vi "Set Settings.vi"(8 "error in (no error)":errorcluster, 10 "Settings":T1, 11 "Acrobat Template in":refnum<class "Application.lvclass">) -> (0 "error out":errorcluster, 3 "Acrobat Template out":refnum<class "Application.lvclass">)   [LabVIEW 2017, in "Application.lvlib" / "Application.lvclass"]
uses:
  Application.lvclass
  Settings/Class Settings -- Cluster.ctl
  <vilib>/TSS/ACRObat Test Framework/Classes/Data/Data Viewer/Settings/Pass Fail Criteria -- Cluster.ctl
  Application.lvclass/Application.ctl
  Settings/App Settings.lvclass
  <vilib>/TSS/ACRObat Test Framework/Classes/Data/Data Viewer/Settings/Data Viewer Settings.lvclass
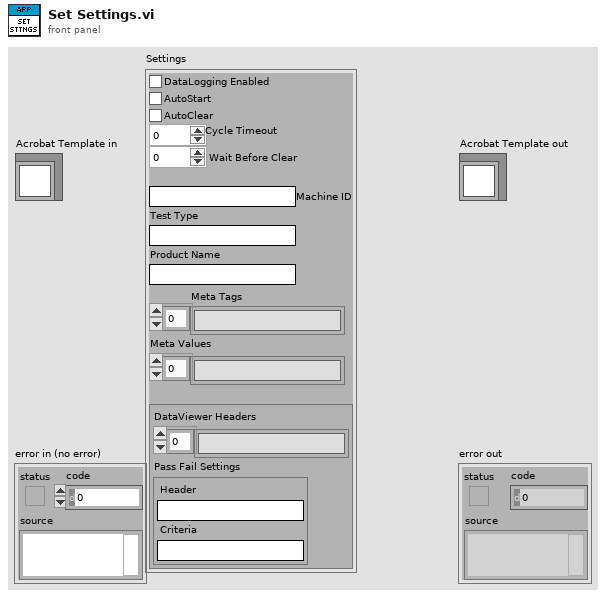
[diagram p1: front panel]
types:
  T1 = typedef "Application.lvlib/App Settings.lvclass/Class Settings -- Cluster.ctl" = cluster{"DataLogging Enabled":bool, "AutoStart":bool, "AutoClear":bool, "Cycle Timeout":u32, "Wait Before Clear":u32, "Machine ID":string, "Test Type":string, "Product Name":string, "Meta Tags":string[], "Meta Values":string[], "Viewer Settings":cluster{"DataViewer Headers":string[], "Pass Fail Settings":T2}}
  T2 = typedef "Data Viewer.lvlib/Data Viewer Settings.lvclass/Pass Fail Criteria -- Cluster.ctl" = cluster{"Header":string, "Criteria":string}
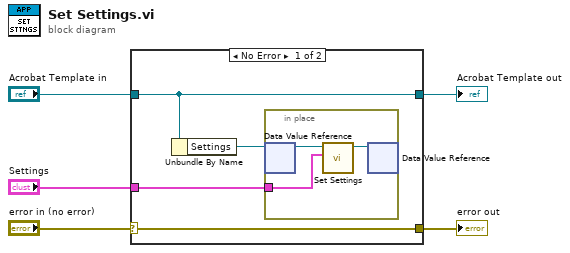
[diagram p0: block diagram]
diagram:
  n1 = case shown="No Error" "error in (no error)" {
    selector: "error in (no error)" -> [w9 w14]
    tunnel: [w9 w14] -> w4
    tunnel: [w8 w13] -> w2
    tunnel: "Acrobat Template in" -> [w8 w13]
    tunnel: "Settings" -> [w6 _]
    frame No Error {
      n2 = Unbundle By Name(w8) -> ("Settings"=w7:refnum<data-value>)
      n3 = in-place {
        in-place-border: w6 -> [w10]
        n4 = in-place-dvr #1(w7) -> (w12:refnum<class "App Settings.lvclass">)  [unwired: 1 out]
        n5 = call-dynamic "Set Settings.vi"("Settings"=w10, "App Settings in"=w12) -> ("App Settings out"=w11:refnum<class "App Settings.lvclass">)  [unwired: 8 in, 1 out]
        n6 = in-place-dvr #1(w11) -> ()  [unwired: 2 out]
      }
    }
    frame Error {
    }
  }
  "error out" <- w4
  "Acrobat Template out" <- w2
